vi "Revision Query.vi"(8 "error in (no error)":errorcluster, 11 "VISA resource name":refnum<visa-resource-name>) -> (0 "error out":errorcluster, 1 "Instrument Firmware Revision":string, 2 "Instrument Driver Revision":string, 3 "VISA resource name out":refnum<visa-resource-name>)   [LabVIEW 2014, in "Associated Research SC6540.lvlib"]
doc: "Query the current instrument firmware revision and instrument driver revision.\n\nRefer to the Readme file for detailed driver information including modification history."
uses:
  <instrlib>/Associated Research SC6540/Associated Research SC6540.lvlib
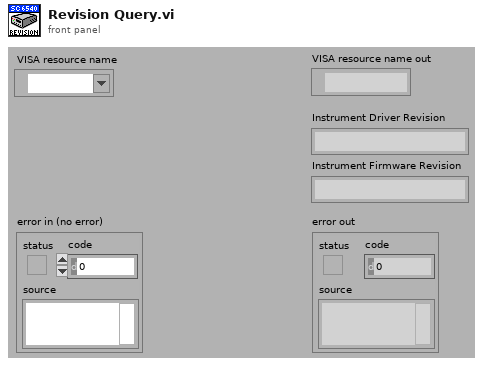
[diagram p1: front panel]
types:
  T1 = enum32{"invalid app kind", "Development System", "Run Time System", "Student Edition", "Embedded LabVIEW", "Evaluation", "Custom"}
  T2 = cluster{"Major":u16, "Minor":u16, "Fix":u16, "Build":u16}
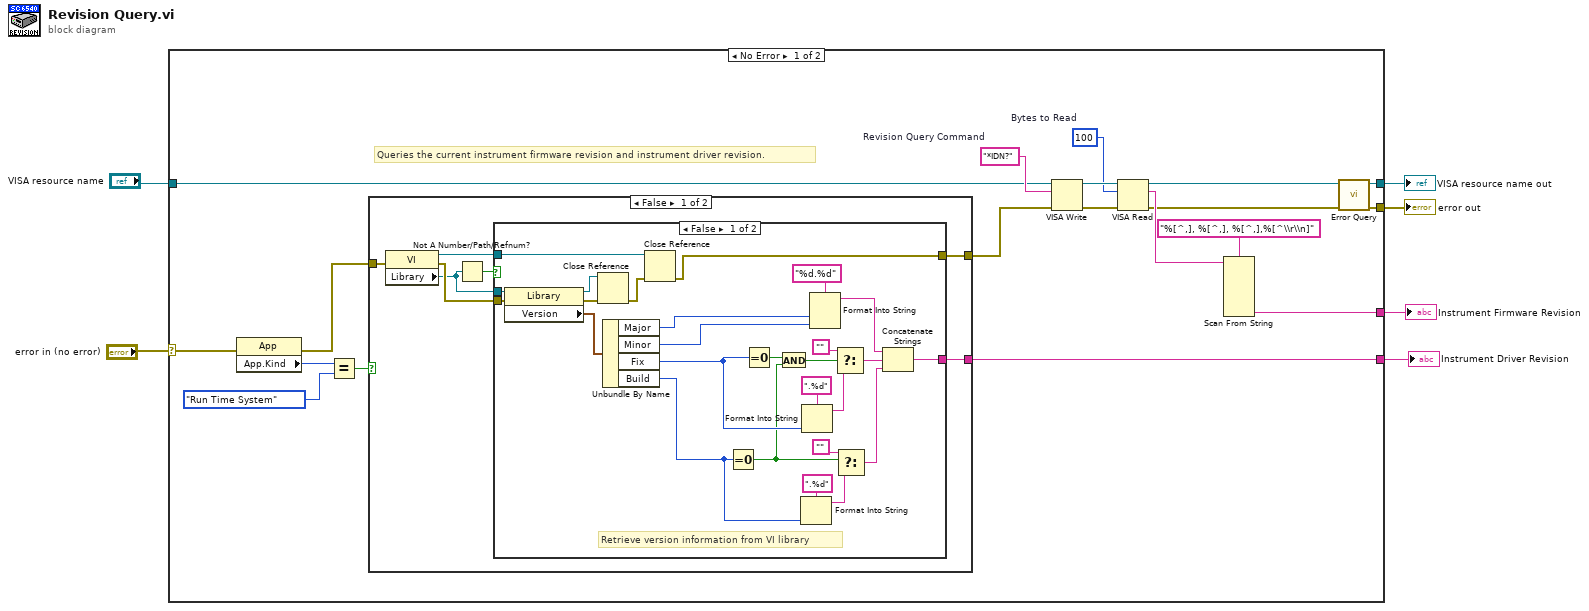
[diagram p0: block diagram]
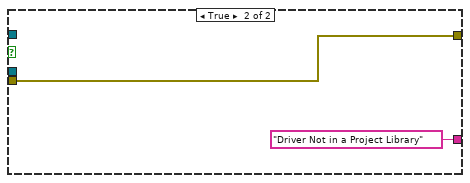
[diagram p2: hidden frame]
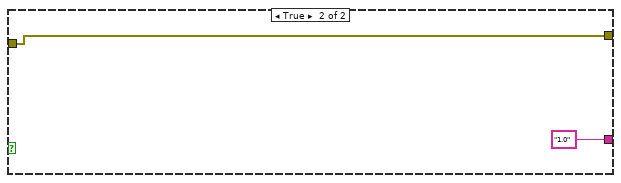
[diagram p3: hidden frame]
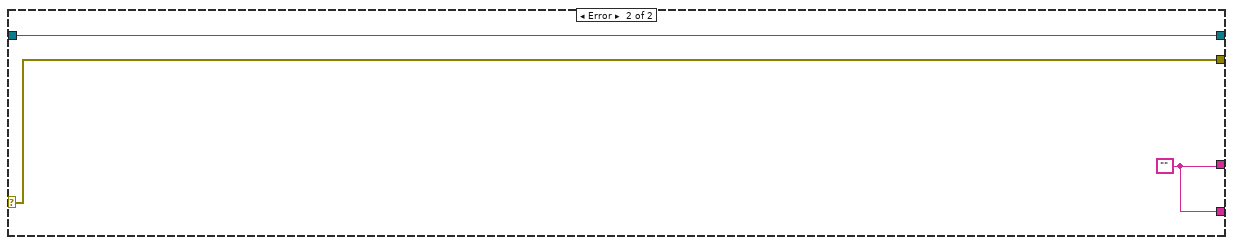
[diagram p4: hidden frame]
diagram:
  n1 = case shown="No Error" "error in (no error)" {
    selector: "error in (no error)" -> [w11 w64]
    tunnel: [w16 w65] -> w6
    tunnel: [w14 w64] -> w5
    tunnel: "VISA resource name" -> [w9 w65]
    tunnel: [w8 w63] -> w2
    tunnel: [w7 w63] -> w1
    frame No Error {
      w13 = "*IDN?"  # Revision Query Command
      w12 = u32 100  # Bytes to Read
      # "Queries the current instrument firmware revision and instrument driver revision."
      n2 = property class="App"(error in=w11) -> (error out=w10:errorcluster, "App.Kind"=w21:T1)  [unwired: 1 in, 1 out]
      n3 = Equal?(x=w21, y=T1."Run Time System" ("Application:Kind")) -> (x = y?=w22:bool)
      n4 = case shown="False" w22 {
        tunnel: [w28 "1.0"] -> w7
        tunnel: w10 -> [w27 w61]
        tunnel: [w26 w61] -> w19
        frame False {
          n5 = property class="VI"(error in=w27) -> (reference out=w32:refnum<vi>, error out=w31:errorcluster, "Library"=w30:refnum<vi>)  [unwired: 1 in]
          n6 = Not A Number/Path/Refnum?(number/path/refnum=w30) -> (NaN/Path/Refnum?=w29:bool)
          n7 = case shown="False" w29 {
            tunnel: w32 -> [w55 _]
            tunnel: w31 -> [w40 w60]
            tunnel: [w35 w60] -> w26
            tunnel: [w34 "Driver Not in a Project Library"] -> w28
            tunnel: w30 -> [w33 _]
            frame False {
              # "Retrieve version information from VI library"
              n8 = property class="Library"(reference=w33, error in=w40) -> (reference out=w57:refnum<vi>, error out=w58:errorcluster, "Version"=w54:T2)
              n9 = Close Reference(reference=w57, error in (no error)=w58) -> (error out=w56:errorcluster)
              n10 = Unbundle By Name(w54) -> ("Major"=w43:u16, "Minor"=w42:u16, "Fix"=w39:u16, "Build"=w41:u16)
              n11 = Close Reference(reference=w55, error in (no error)=w56) -> (error out=w35:errorcluster)
              n12 = Equal To 0?(x=w41) -> (x = 0?=w37:bool)
              n13 = Equal To 0?(x=w39) -> (x = 0?=w38:bool)
              n14 = And(x=w38, y=w37) -> (x .and. y?=w36:bool)
              n15 = Format Into String(format string=".%d", w41) -> (resulting string=w47:string)  [unwired: 2 in, 1 out]
              n16 = Format Into String(format string=".%d", w39) -> (resulting string=w51:string)  [unwired: 2 in, 1 out]
              n17 = Format Into String(format string="%d.%d", w43, w42) -> (resulting string=w49:string)  [unwired: 2 in, 1 out]
              n18 = Select(t="", s=w36, f=w51) -> (s? t:f=w48:string)
              n19 = Select(t="", s=w37, f=w47) -> (s? t:f=w44:string)
              n20 = Concatenate Strings(w49, w48, w44) -> (w34:string)
            }
            frame True {
            }
          }
        }
        frame True {
        }
      }
      n21 = VISA Write(VISA resource name=w9, write buffer=w13, error in (no error)=w19) -> (VISA resource name out=w25:refnum<visa-resource-name>, error out=w23:errorcluster)  [unwired: 1 out]
      n22 = VISA Read(VISA resource name=w25, byte count=w12, error in (no error)=w23) -> (VISA resource name out=w24:refnum<visa-resource-name>, read buffer=w17:string, error out=w15:errorcluster)  [unwired: 1 out]
      n23 = Scan From String(format string="%[^,], %[^,], %[^,],%[^\\r\\n]", input string=w17) -> (output 4=w8:string)  [unwired: 9 in, 3 out]
      n24 = call <instrlib>:"Error Query.vi"("error in (no error)"=w15, "VISA resource name"=w24) -> ("error out"=w14:errorcluster, "VISA resource name out"=w16:refnum<visa-resource-name>)  [unwired: 6 in, 2 out]
    }
    frame Error {
      w63 = ""
    }
  }
  "error out" <- w5
  "VISA resource name out" <- w6
  "Instrument Firmware Revision" <- w2
  "Instrument Driver Revision" <- w1
